vi "Handle Errors.vi"(8 "error in":errorcluster, 11 "nCRD in":refnum<class "nCRD.lvclass">) -> (0 "error out":errorcluster, 2 "errors":errorcluster[](array[cluster]), 3 "nCRD out":refnum<class "nCRD.lvclass">)   [LabVIEW 2015, in "nCRD.lvclass"]
uses:
  nCRD.lvclass
  Reusable/CRDS/Main/CRDS.lvclass
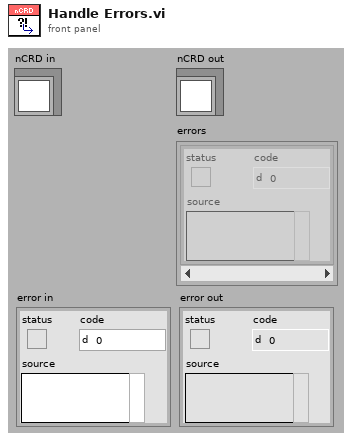
[diagram p1: front panel]
types:
  T1 = typedef "FPGA Ref.ctl" = refnum<k20>
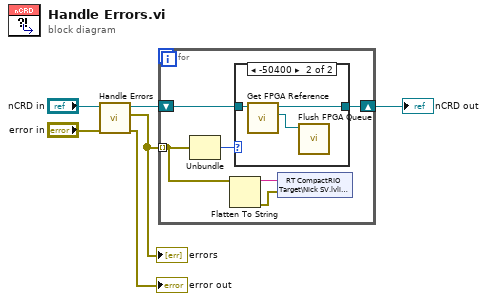
[diagram p0: block diagram]
diagram:
  n1 = call-parent "Handle Errors.vi"("error in"="error in", "Instrument in"="nCRD in") -> ("error out"=→"error out":errorcluster, "errors"=w3:errorcluster[], "Instrument out"=w2:refnum<class "nCRD.lvclass">)  [unwired: 7 in]
  "errors" <- w3
  n2 = for {
    tunnel: w3 -> [w10] mode=indexing
    shift-right: [w7] -> w1
    shift-left: w2 -> [w8]
    n3 = Unbundle(w10) -> ("code"=w9:i32)  [unwired: 2 out]
    n4 = Flatten To String(anything=w10) -> (data string=w12:string, error out=w11:errorcluster)  [unwired: 3 in, 1 out]
    n5 = case shown="-50400" w9 {
      tunnel: w8 -> [w13 w16]
      tunnel: [w13 w15] -> w7
      frame 0, Default {
      }
      frame -50400 {
        n6 = call "Get FPGA Reference.vi"("nCRD in"=w16) -> ("Accessors:FPGA Ref"=w14:T1, "nCRD Out"=w15:refnum<class "nCRD.lvclass">)  [unwired: 8 in, 1 out]
        n7 = call "Flush FPGA Queue.vi"("Refnum in"=w14) -> ()  [unwired: 10 in, 1 out]
      }
    }
    n8 = shared-variable "RT CompactRIO Target\\Nick SV.lvlib\\Errors"(w12, error in=w11) -> ()  [unwired: 1 out]
  }
  "nCRD out" <- w1
